vi "Fast_string_Replace.vi"(2 "mode":enum16{"simple", "regex"}(ring)=enum."regex", 3 "Replace match with:":string, 4 "Input String":string, 5 "matchThis":string) -> (0 "Number Found":i32, 1 "Output String":string)   [LabVIEW 2022 SP3]
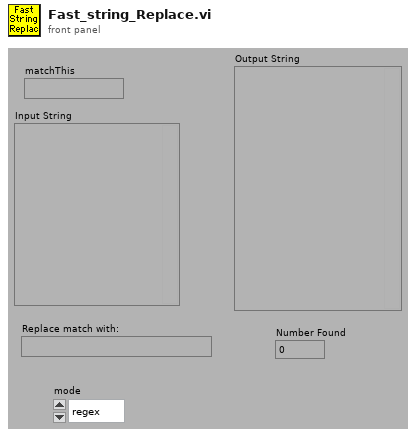
[diagram p1: front panel]
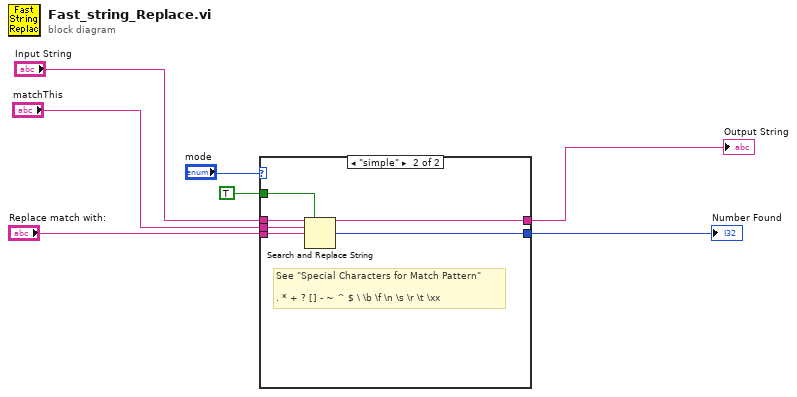
[diagram p0: block diagram]
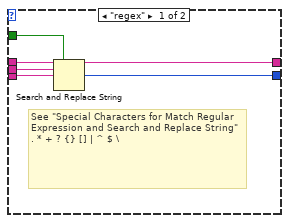
[diagram p2: hidden frame]
diagram:
  n1 = case shown="\"simple\"" "mode" {
    tunnel: "Input String" -> [w13 w19]
    tunnel: "Replace match with:" -> [w12 w18]
    tunnel: "matchThis" -> [w11 w17]
    tunnel: TRUE ("replace all? (F)") -> [w10 w16]
    tunnel: [w9 w15] -> w3
    tunnel: [w8 w14] -> w2
    frame "regex" {
      # "See \"Special Characters for Match Regular Expression and Search and Replace String\"\n. * + ? {} [] | ^ $ \\"
      n2 = Search and Replace String(replace all?=w10, input string=w13, search string=w11, replace string=w12) -> (result string=w8:string, number of replacements=w9:i32)  [unwired: 4 in, 2 out]
    }
    frame "simple" {
      # "See \"Special Characters for Match Pattern\"\n\n. * + ? [] - ~ ^ $ \\ \\b \\f \\n \\s \\r \\t \\xx"
      n3 = Search and Replace String(replace all?=w16, input string=w19, search string=w17, replace string=w18) -> (result string=w14:string, number of replacements=w15:i32)  [unwired: 4 in, 2 out]
    }
  }
  "Output String" <- w2
  "Number Found" <- w3
